vi "Konvolucio MCAN120803 Example_0006 Read.vi"() -> ()   [LabVIEW 2011]
uses:
  <instrlib>/Konvolucio MCAN120803/Types/MessageType.ctl
  <instrlib>/Konvolucio MCAN120803/Public/Attributes/AttrSetTermination.vi
  <instrlib>/Konvolucio MCAN120803/Public/Attributes/AttrGetRxPendingMsg.vi
  <instrlib>/Konvolucio MCAN120803/Konvolucio MCAN120803.lvlib
panel:
  out "Messages":T1[](array[typedef])
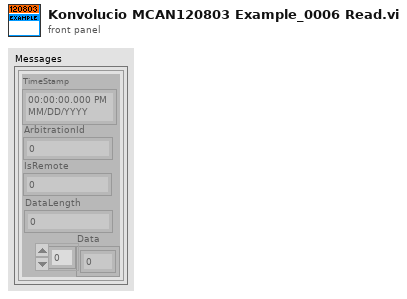
[diagram p1: front panel]
types:
  T1 = typedef "Konvolucio MCAN120803.lvlib/MessageType.ctl" = cluster{"TimeStamp":timestamp, "ArbitrationId":u32, "IsRemote":u8, "DataLength":u8, "Data":u8[]}
  T2 = typedef "Konvolucio MCAN120803.lvlib/CanHandleType.ctl" = cluster{"AdapterDevice":refnum<k24>}
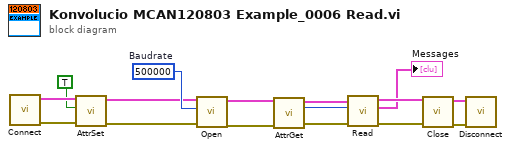
[diagram p0: block diagram]
diagram:
  w16 = u32 500000  # Baudrate
  n1 = call <instrlib>:"Connect.vi"() -> ("error out"=w15:errorcluster, "CanHandleOut"=w13:T2)  [unwired: 10 in]
  n2 = call-poly <instrlib>:"AttrSet.vi"("error in"=w15, "Enabled"=TRUE, "CanHandleIn"=w13) -> ("error out"=w14:errorcluster, "CanHandleOut"=w12:T2)  [unwired: 6 in]
  n3 = call <instrlib>:"Open.vi"("error in"=w14, "Baudrate"=w16, "CanHandleIn"=w12) -> ("error out"=w8:errorcluster, "CanHandleOut"=w7:T2)  [unwired: 7 in]
  n4 = call-poly <instrlib>:"AttrGet.vi"("error in"=w8, "CanHandleIn"=w7) -> ("error out"=w6:errorcluster, "Value"=w4:i32, "CanHandleOut"=w5:T2)  [unwired: 7 in]
  n5 = call <instrlib>:"Read.vi"("error in"=w6, "Request Number of Message"=w4, "CanHandleIn"=w5) -> ("error out"=w3:errorcluster, "Messages"=→"Messages":T1[], "CanHandleOut"=w2:T2)  [unwired: 6 in]
  n6 = call <instrlib>:"Close.vi"("error in"=w3, "CanHandleIn"=w2) -> ("error out"=w10:errorcluster, "CanHandleOut"=w9:T2)  [unwired: 8 in]
  n7 = call <instrlib>:"Disconnect.vi"("error in"=w10, "CanHandleIn"=w9) -> ()  [unwired: 9 in, 1 out]
